vi "Step Flow.vi"(8 "error in (no error)":errorcluster, 11 "String Compare in":refnum<class "String Compare.lvclass">) -> (0 "error out":errorcluster, 3 "String Compare out":refnum<class "String Compare.lvclass">)   [LabVIEW 2015, in "String Compare.lvclass"]
uses:
  String Compare.lvclass
  classes/Step/Execution/StepState.ctl
  classes/Step/Execution/Step State Enum.ctl
  classes/Step/Execution/Step Flow Control.ctl
  classes/Step/Execution/Step.lvclass
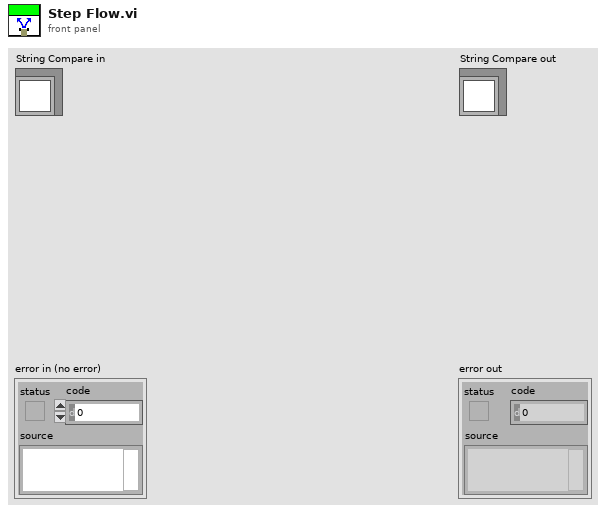
[diagram p1: front panel]
types:
  T1 = typedef "Step.lvclass/StepState.ctl" = cluster{"Step State":T2, "Flow Control":T3, "Jump Index":i32, "Done":bool}
  T2 = typedef "Step.lvclass/Step State Enum.ctl" = enum16{"Start", "Skipped", "Timeout", "Completed", "Running", "Aborted"}
  T3 = typedef "Step.lvclass/Step Flow Control.ctl" = enum16{"Next Step", "Jump"}
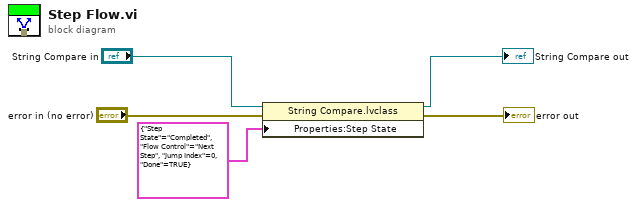
[diagram p0: block diagram]
diagram:
  n1 = property class="String Compare.lvclass"(reference="String Compare in", error in="error in (no error)", "Properties:Step State"=T1 {"Step State"=enum."Completed", "Flow Control"=enum."Next Step", "Jump Index"=0, "Done"=TRUE} ("Step State")) -> (reference out=→"String Compare out":refnum<class "String Compare.lvclass">, error out=→"error out":errorcluster)
